vi "Assign Pixel to Wing Sector (Host).vi"(6 "Pixel Intensity In":u8, 7 "Right Wing?":bool, 8 "Sector Parameters":T1, 9 "Pixel Y":u16, 10 "Pixel X":u16) -> (0 "Pixel Y Out":u16, 1 "Pixel Intensity Out":u8, 2 "sector #":u8, 3 "output valid":bool, 4 "Pixel X Out":u16)   [LabVIEW 2013]
uses:
  FPGA/Sector/Accumulate/Sector Parameter Cluster.ctl
  <vilib>/rvi/FXPMathLib/FxpRectToPolar/subVIs/nifxpmath_RectToPolar_SimConfig.ctl
  <vilib>/rvi/FXPMathLib/FxpDiv/subVIs/nifxpmath_Div_SimConfig.ctl
  <vilib>/rvi/FXPMathLib/FxpRectToPolar/simVIs/DllFxpRectToPolarTemp_sub.vi
  <vilib>/rvi/FXPMathLib/FxpDiv/simVIs/DllFxpDivTemp_sub.vi
  <vilib>/rvi/FXPMathLib/FxpSub/XNode/nifxpmath_Sub.xnode
  <vilib>/rvi/FXPMathLib/FxpRectToPolar/XNode/nifxpmath_RectToPolar.xnode
  <vilib>/rvi/FXPMathLib/FxpAdd/XNode/nifxpmath_Add.xnode
  <vilib>/rvi/FXPMathLib/FxpDiv/XNode/nifxpmath_Div.xnode
  <vilib>/rvi/FXPMathLib/sim/FxpSim.dll
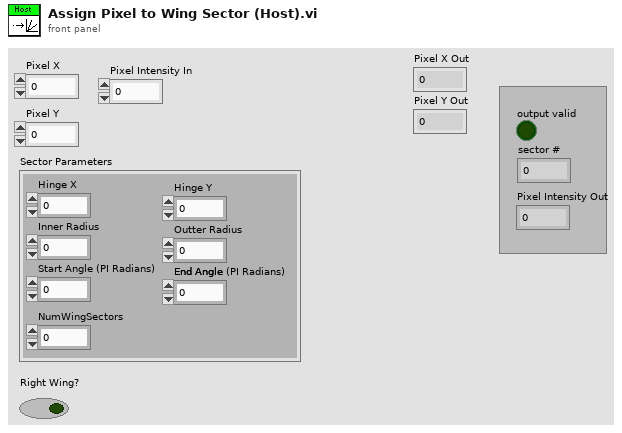
[diagram p1: front panel]
types:
  T1 = typedef "Sector Parameter Cluster.ctl" = cluster{"Start Angle":fxp<+,17,3>, "End Angle":fxp<+,17,3>, "Inner Radius":u16, "Outter Radius":u16, "Hinge X":u16, "Hinge Y":u16, "NumWingSectors":u8}
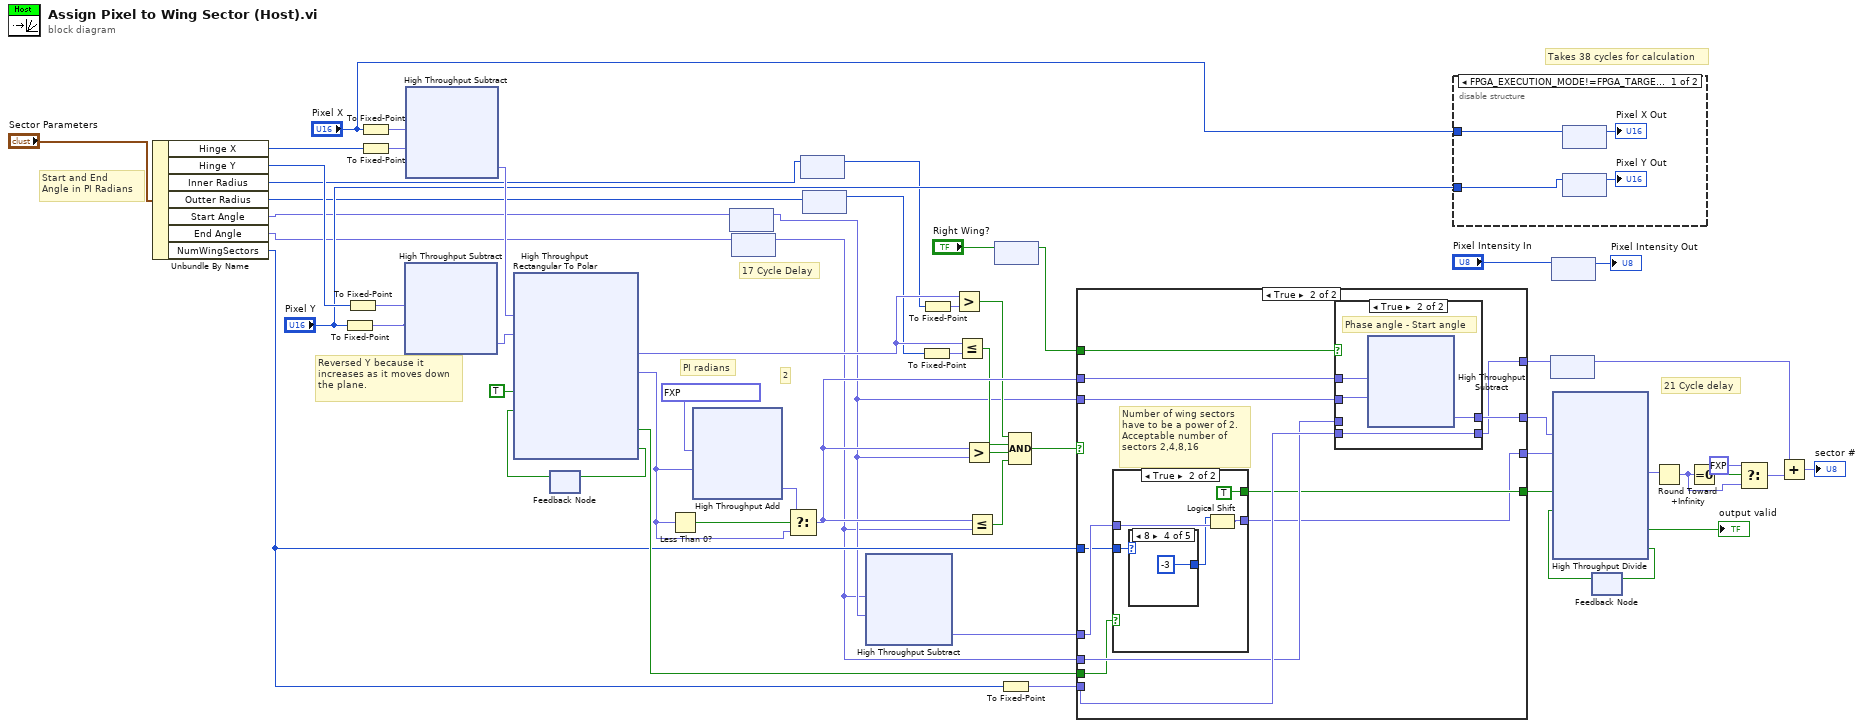
[diagram p0: block diagram]
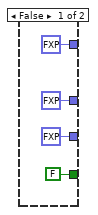
[diagram p3: hidden frame]
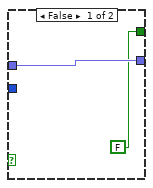
[diagram p4: hidden frame]
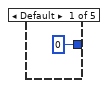
[diagram p5: hidden frame]
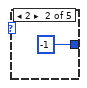
[diagram p6: hidden frame]
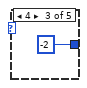
[diagram p7: hidden frame]
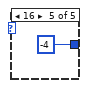
[diagram p8: hidden frame]
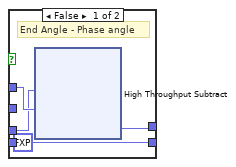
[diagram p9: hidden frame]
diagram:
  # "Takes 38 cycles for calculation"
  # "17 Cycle Delay"
  # "Reversed Y because it\nincreases as it moves down\nthe plane."
  # "PI radians"
  # "21 Cycle delay"
  # "Start and End\nAngle in PI Radians"
  # "2"
  n1 = Unbundle By Name("Sector Parameters") -> ("Hinge X"=w19:u16, "Hinge Y"=w41:u16, "Inner Radius"=w13:u16, "Outter Radius"=w11:u16, "Start Angle"=w9:fxp<+,17,3>, "End Angle"=w7:fxp<+,17,3>, "NumWingSectors"=w24:u8)
  n2 = To Fixed-Point(number="Pixel Y") -> (fixed-point=w29:fxp<+,11,11>)  [unwired: 1 in]
  n3 = To Fixed-Point(number=w41) -> (fixed-point=w30:fxp<+,11,11>)  [unwired: 1 in]
  n4 = To Fixed-Point(number="Pixel X") -> (fixed-point=w28:fxp<+,11,11>)  [unwired: 1 in]
  n5 = To Fixed-Point(number=w19) -> (fixed-point=w27:fxp<+,11,11>)  [unwired: 1 in]
  n6 = xnode "High Throughput Subtract"("x"=w30, "y"=w29) -> ("x-y"=w39:fxp<+/-,12,12>)
  n7 = xnode "High Throughput Subtract"("x"=w28, "y"=w27) -> ("x-y"=w38:fxp<+/-,12,12>)
  n8 = feedback #1() -> (w46:bool)  [unwired: 1 in]
  n9 = xnode "High Throughput Rectangular To Polar"("x"=w38, "y"=w39, "input valid"=TRUE, "ready for output (T)"=w46) -> ("magnitude"=w56:fxp<+,12,12>, "phase (pi)"=w52:fxp<+/-,16,2>, "output valid"=w25:bool, "ready for input"=w47:bool)
  n10 = feedback-in #1(w47) -> ()
  n11 = Less Than 0?(x=w52) -> (x < 0?=w53:bool)
  n12 = xnode ("High Throughput Add")("x"=fxp<+/-,16,2> 1.99993896484375 ("y"), "y"=w52) -> ("x+y"=w51:fxp<+/-,17,3>)
  n13 = feedback #2() -> (w8:fxp<+,17,3>)  [unwired: 1 in]
  n14 = feedback-in #2(w9) -> ()
  n15 = feedback #3() -> (w6:fxp<+,17,3>)  [unwired: 1 in]
  n16 = feedback-in #3(w7) -> ()
  n17 = Select(t=w51, s=w53, f=w52) -> (s? t:f=w49:fxp<+/-,17,3>)
  n18 = feedback #4() -> (w12:u16)  [unwired: 1 in]
  n19 = feedback-in #4(w13) -> ()
  n20 = feedback #5() -> (w10:u16)  [unwired: 1 in]
  n21 = feedback-in #5(w11) -> ()
  n22 = xnode ("High Throughput Subtract")("x"=w6, "y"=w8) -> ("x-y"=w26:fxp<+/-,17,6>)
  n23 = To Fixed-Point(number=w10) -> (fixed-point=w55:fxp<+,16,16>)  [unwired: 1 in]
  n24 = To Fixed-Point(number=w12) -> (fixed-point=w57:fxp<+,16,16>)  [unwired: 1 in]
  n25 = Greater?(x=w56, y=w57) -> (0:w45:bool)
  n26 = Less Or Equal?(x=w56, y=w55) -> (x <= y?=w44:bool)
  n27 = Greater?(x=w49, y=w8) -> (0:w43:bool)
  n28 = Less Or Equal?(x=w49, y=w6) -> (x <= y?=w42:bool)
  n29 = feedback #6() -> (w17:bool)  [unwired: 1 in]
  n30 = feedback-in #6("Right Wing?") -> ()
  n31 = To Fixed-Point(number=w24) -> (fixed-point=w40:fxp<+,8,8>)  [unwired: 1 in]
  n32 = Compound Arithmetic op=AND(w45, w44, w43, w42) -> (w54:bool)
  n33 = case shown="True" w54 {
    tunnel: w49 -> [_ w73]
    tunnel: w8 -> [_ w72]
    tunnel: [fxp<+/-,17,6> 0.0 ("x-y") w63] -> w34
    tunnel: w6 -> [_ w70]
    tunnel: w40 -> [_ w71]
    tunnel: [fxp<+/-,19,5> 0.0 ("x-y") w69] -> w35
    tunnel: [FALSE ("output valid") w64] -> w33
    tunnel: [fxp<+,8,8> 0.0 w68] -> w31
    tunnel: w26 -> [_ w67]
    tunnel: w25 -> [_ w66]
    tunnel: w24 -> [_ w65]
    tunnel: w17 -> [_ w62]
    frame False {
    }
    frame True {
      # "Number of wing sectors\nhave to be a power of 2.\nAcceptable number of\nsectors 2,4,8,16"
      n34 = case shown="True" w66 {
        tunnel: w65 -> [_ w80]
        tunnel: w67 -> [w75 w79]
        tunnel: [w75 w77] -> w63
        tunnel: [FALSE ("output valid") TRUE ("output valid")] -> w64
        frame False {
        }
        frame True {
          n35 = case shown="8" w80 {
            tunnel: [i16 0 ("y") i16 -1 ("y") i16 -2 ("y") i16 -3 ("y") i16 -4 ("y")] -> w78
            frame Default {
            }
            frame 2 {
            }
            frame 4 {
            }
            frame 8 {
            }
            frame 16 {
            }
          }
          n36 = Logical Shift(y=w78, x=w79) -> (x << y=w77:fxp<+/-,17,6>)
        }
      }
      n37 = case shown="True" w62 {
        tunnel: w73 -> [w88 w93]
        tunnel: w72 -> [_ w92]
        tunnel: [w89 w91] -> w69
        tunnel: w71 -> [_ w90]
        tunnel: [fxp<+,8,8> 0.0 w90] -> w68
        tunnel: w70 -> [w87 _]
        frame False {
          # "End Angle - Phase angle"
          n38 = xnode "High Throughput Subtract"("x"=w87, "y"=w88) -> ("x-y"=w89:fxp<+/-,19,5>)
        }
        frame True {
          # "Phase angle - Start angle"
          n39 = xnode ("High Throughput Subtract")("x"=w93, "y"=w92) -> ("x-y"=w91:fxp<+/-,19,5>)
        }
      }
    }
  }
  n40 = disable-structure shown="FPGA_EXECUTION_MODE!=FPGA_TARGET" {
    disable-tunnel: "Pixel X" -> [w97 _]
    disable-tunnel: "Pixel Y" -> [w96 _]
    frame condition #0 (active) {
      n41 = feedback #7() -> (→"Pixel X Out":u16)  [unwired: 1 in]
      n42 = feedback-in #7(w97) -> ()
      n43 = feedback #8() -> (→"Pixel Y Out":u16)  [unwired: 1 in]
      n44 = feedback-in #8(w96) -> ()
    }
    frame condition #1 {
    }
  }
  n45 = feedback #9() -> (w3:fxp<+,8,8>)  [unwired: 1 in]
  n46 = feedback-in #9(w31) -> ()
  n47 = feedback #10() -> (→"Pixel Intensity Out":u8)  [unwired: 1 in]
  n48 = feedback-in #10("Pixel Intensity In") -> ()
  n49 = feedback #11() -> (w32:bool)  [unwired: 1 in]
  n50 = xnode "High Throughput Divide"("x"=w35, "y"=w34, "input valid"=w33, "ready for output (T)"=w32) -> ("x/y"=w16:fxp<+/-,19,16>, "output valid"=→"output valid":bool, "ready for input"=w37:bool)
  n51 = feedback-in #11(w37) -> ()
  n52 = Round Toward +Infinity(x=w16) -> (ceil(x): smallest int >= x=w15:fxp<+/-,17,17>)
  n53 = Equal To 0?(x=w15) -> (x = 0?=w2:bool)
  n54 = Select(t=fxp<+/-,17,17> 1.0, s=w2, f=w15) -> (s? t:f=w5:fxp<+/-,17,17>)
  n55 = Add(x=w3, y=w5) -> (x+y=→"sector #":fxp<+/-,17,17>)
